vi "Sample_Finite_PulseTrigger.vi"() -> ()   [LabVIEW 2013]
doc: "This samples demonstrates how to sample a finite waveform."
uses:
  <userlib>/ArtScope/Trigger/ArtScope_ConfigureTriggerPulse.vi
  <userlib>/ArtScope/Fetch/ArtScope_FetchBinary8.vi
  <userlib>/ArtScope/_SubVI/ArtScope_ArrayByChannel_U8.vi
panel:
  in  "slope":i32(ring) items=["Greater", "Less", "Equal", "Nequal"]
  out "error out":errorcluster
  in  "reference position":dbl
  in  "width(ns)":i32
  in  "sensitive(ns)":i32
  in  "polarity":i32(ring) items=["Positive", "Negative"]
  in  "level(mV)":dbl
  in  "count":i32=1
  in  "source":string(combo)="VAL_TRIGGER_ATR"
  in  "range(Vpp)":i32(ring) items=["20V", "10V", "2V", "40V", "16V", "8V", "4V", "1.6V", "800m", "400m", "160m", "80m", "40m"]
  in  "offset(mV)":i32
  in  "num samples":i32=1000
  in  "Stop":bool
  out "waveform":u8[][](graph)
  in  "timeout(s)":dbl=10.0
  in  "min record length":i32=6000
  in  "min sample rate":dbl=800000.0
  in  "coupling":i32(ring) items=["DC", "AC"]
  in  "channel name":string="0"
  in  "resource name":string="Dev1"
  # "Vertical"
  # "Horizontal"
  # "Trigger"
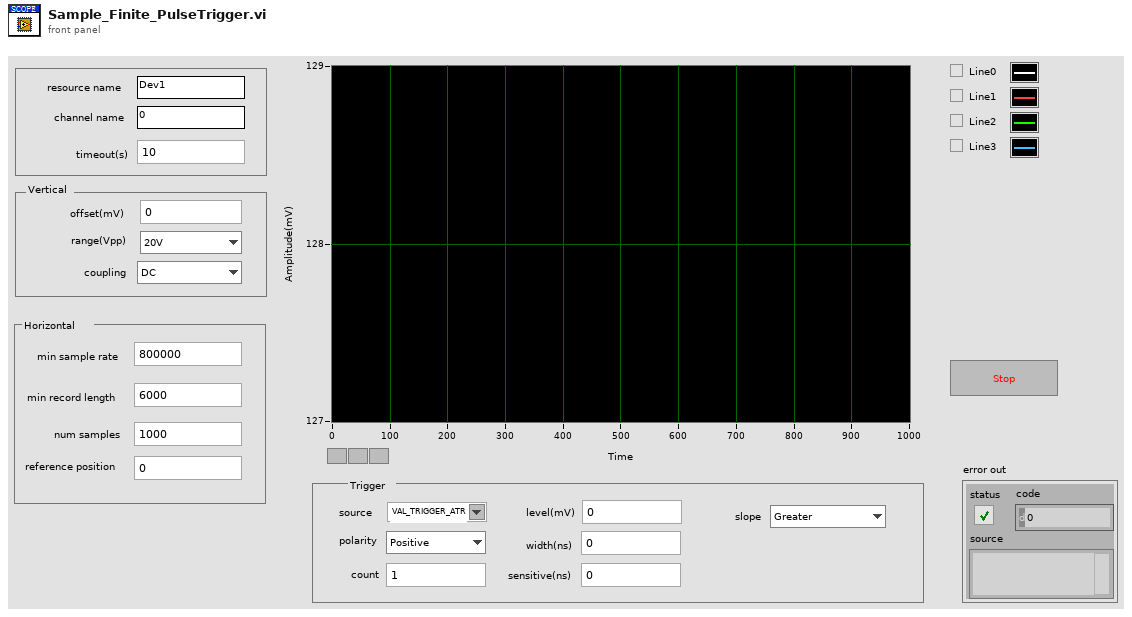
[diagram p1: front panel]
types:
  T1 = cluster{"fLSB":cluster{dbl, dbl, dbl, dbl, dbl, dbl, dbl, dbl}, "RangeValue":cluster{dbl, dbl, dbl, dbl, dbl, dbl, dbl, dbl}, "wMaxLSB":u32, "TriggerMode":i32, "sampLengthPerChan":u32, "pAvailSampsPoints":u32, "channelCount":i32}
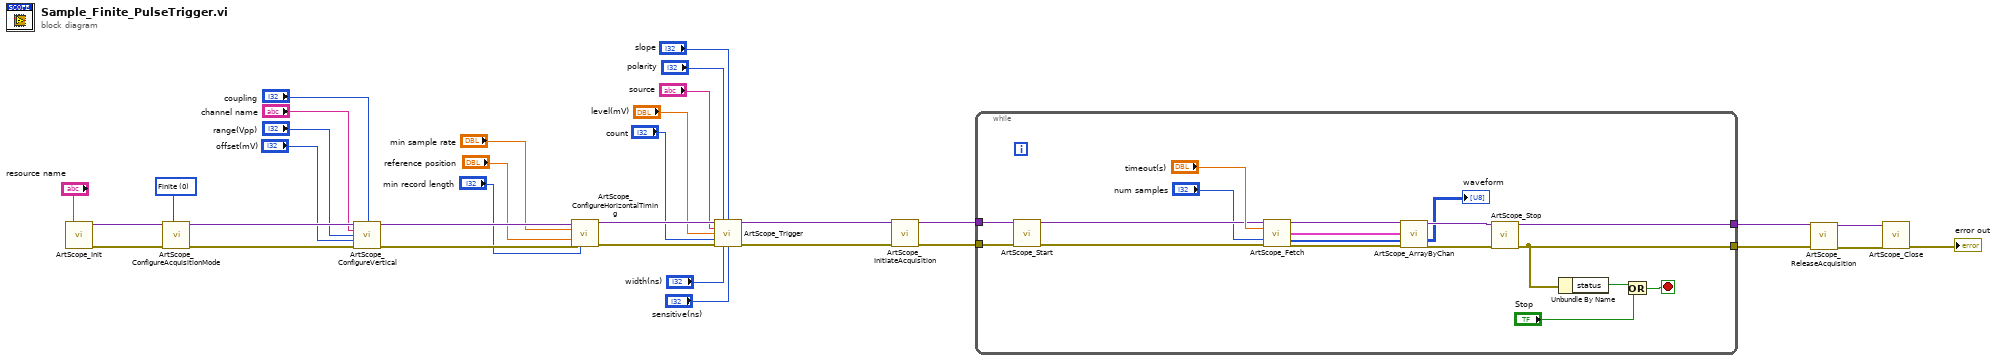
[diagram p0: block diagram]
diagram:
  w26 = 0 items=["Finite", "Continuous"] ("AcuqMode")
  n1 = call <userlib>:"ArtScope_Init.vi"("task name"="resource name") -> ("task handle"=w27:variant, "error out"=w28:errorcluster)  [unwired: 13 in]
  n2 = call <userlib>:"ArtScope_ConfigureAcquisitionMode.vi"("task handle"=w27, "acquisition mode"=w26, "error in (no error)"=w28) -> ("task handle"=w25:variant, "error out"=w29:errorcluster)  [unwired: 11 in]
  n3 = call <userlib>:"ArtScope_ConfigureVertical.vi"("task handle"=w25, "coupling"="coupling", "channels"="channel name", "range(Vpp)"="range(Vpp)", "offset"="offset(mV)", "error in (no error)"=w29) -> ("task handle"=w31:variant, "error out"=w30:errorcluster)  [unwired: 8 in]
  n4 = call <userlib>:"ArtScope_ConfigureHorizontalTiming.vi"("task handle"=w31, "min sample rate"="min sample rate", "reference position"="reference position", "error in (no error)"=w30, "min record length"="min record length") -> ("task handle"=w23:variant, "error out"=w24:errorcluster)  [unwired: 9 in]
  n5 = call-poly <userlib>:"ArtScope_Trigger.vi"("task handle"=w23, "polarity"="polarity", "slope"="slope", "trigger source"="source", "level"="level(mV)", "trigger count"="count", "error in (no error)"=w24, "width"="width(ns)", "trigger sensitive"="sensitive(ns)") -> ("task handle"=w15:variant, "error out"=w14:errorcluster)  [unwired: 5 in]
  n6 = call <userlib>:"ArtScope_InitiateAcquisition.vi"("task handle"=w15, "error in (no error)"=w14) -> ("task handle"=w13:variant, "error out"=w12:errorcluster)  [unwired: 12 in]
  n7 = while {
    tunnel: [w47] -> w19
    tunnel: [w46] -> w18
    tunnel: w13 -> [w45]
    tunnel: w12 -> [w50]
    stop <- w48 stop-if-true
    n8 = call <userlib>:"ArtScope_Start.vi"("task handle"=w45, "error in (no error)"=w50) -> ("task handle"=w43:variant, "error out"=w42:errorcluster)  [unwired: 12 in]
    n9 = call-poly <userlib>:"ArtScope_Fetch.vi"("task handle"=w43, "timeout"="timeout(s)", "num samples"="num samples", "error in (no error)"=w42) -> ("task handle"=w40:variant, "wfm info"=w36:T1, "data"=w35:u8[], "error out"=w37:errorcluster)  [unwired: 8 in]
    n10 = call-poly <userlib>:"ArtScope_ArrayByChan.vi"("task handle"=w40, "wfm info"=w36, "1D data"=w35, "error in (no error)"=w37) -> ("task handle"=w39:variant, "2D data"=→"waveform":u8[][], "error out"=w38:errorcluster)  [unwired: 9 in]
    n11 = call <userlib>:"ArtScope_Stop.vi"("task handle"=w39, "error in (no error)"=w38) -> ("task handle"=w47:variant, "error out"=w46:errorcluster)  [unwired: 12 in]
    n12 = Unbundle By Name(w46) -> ("status"=w49:bool)
    n13 = Or(x=w49, y="Stop") -> (x .or. y?=w48:bool)
  }
  n14 = call <userlib>:"ArtScope_ReleaseAcquisition.vi"("task handle"=w19, "error in (no error)"=w18) -> ("task handle"=w17:variant, "error out"=w16:errorcluster)  [unwired: 12 in]
  n15 = call <userlib>:"ArtScope_Close.vi"("task handle"=w17, "error in (no error)"=w16) -> ("error out"=→"error out":errorcluster)  [unwired: 13 in]
